vi "Read Rate (Hz).vi"(8 "error in (no error)":errorcluster, 11 "Reset Red Laser Rep Rate in":refnum<class "Reset Red Laser Rep Rate.lvclass">) -> (0 "error out":errorcluster, 2 "Rate (Hz)":i32, 3 "Reset Red Laser Rep Rate out":refnum<class "Reset Red Laser Rep Rate.lvclass">)   [LabVIEW 2014, in "eCRDS Library.lvlib" / "Reset Red Laser Rep Rate.lvclass"]
uses:
  Reset Red Laser Rep Rate.lvclass
  Reset Red Laser Rep Rate.lvclass/Reset Red Laser Rep Rate.ctl
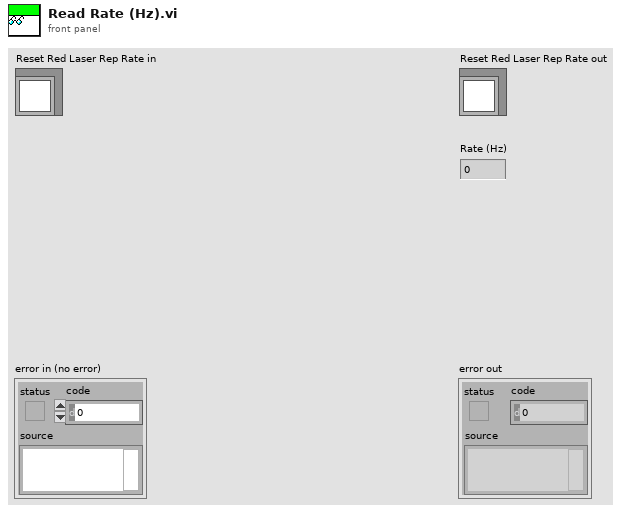
[diagram p1: front panel]
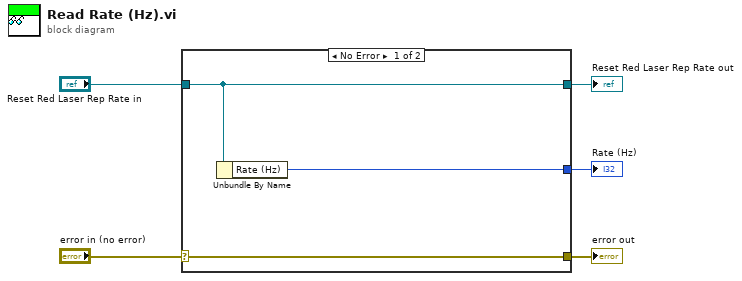
[diagram p0: block diagram]
diagram:
  n1 = case shown="No Error" "error in (no error)" {
    selector: "error in (no error)" -> [w8 w9]
    tunnel: [w8 w9] -> w4
    tunnel: [w7 w10] -> w2
    tunnel: "Reset Red Laser Rep Rate in" -> [w7 w10]
    tunnel: [w6 _] -> w1
    frame No Error {
      n2 = Unbundle By Name(w7) -> ("Rate (Hz)"=w6:i32)
    }
    frame Error {
    }
  }
  "error out" <- w4
  "Reset Red Laser Rep Rate out" <- w2
  "Rate (Hz)" <- w1
